vi "Check Range Hi Press.vi"(0 "reference in":refnum<class "Stand.lvclass">, 1 "init":bool, 11 "error in (no error)":errorcluster) -> (4 "reference out":refnum<class "Stand.lvclass">, 15 "error out":errorcluster)   [LabVIEW 2019, in "Stand.lvclass"]
uses:
  Stand.lvclass
  Stand.lvclass/Stand.ctl
  AI_class/AI.lvclass/AI.ctl
  AnalogComparator_class/AnalogComparator.lvclass/AnalogComparator.ctl
  TypeDef/ExecuteStepState.ctl
  AnalogComparator_class/GetStatus.vi
  AI_class/AI.lvclass
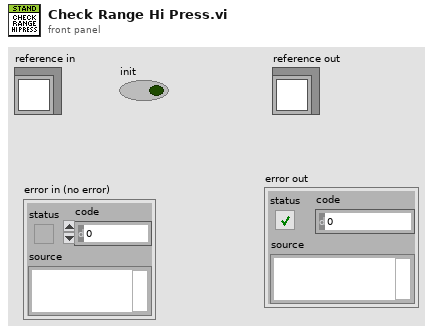
[diagram p1: front panel]
types:
  T1 = typedef "Direction.ctl" = enum8{"DUT", "Chamber"}
  T2 = typedef "AI_Data.ctl" = cluster{"Stat Data":T3, "OutOfRangeMax":bool, "OutOfRangeMin":bool, "HIHI":bool, "HI":bool, "LO":bool, "LOLO":bool}
  T3 = typedef "AI Statistics Data.ctl" = cluster{"raw mean":dbl, "scl mean":dbl, "raw mean 1Hz":dbl, "scl mean 1Hz":dbl}
  T4 = typedef "ExecuteStepState.ctl" = enum16{"Init", "Set: Backpressure ", "Preload: HI", "Set: HI", "Maintenance: HI", "Down: Pressure", "BLOCK"}
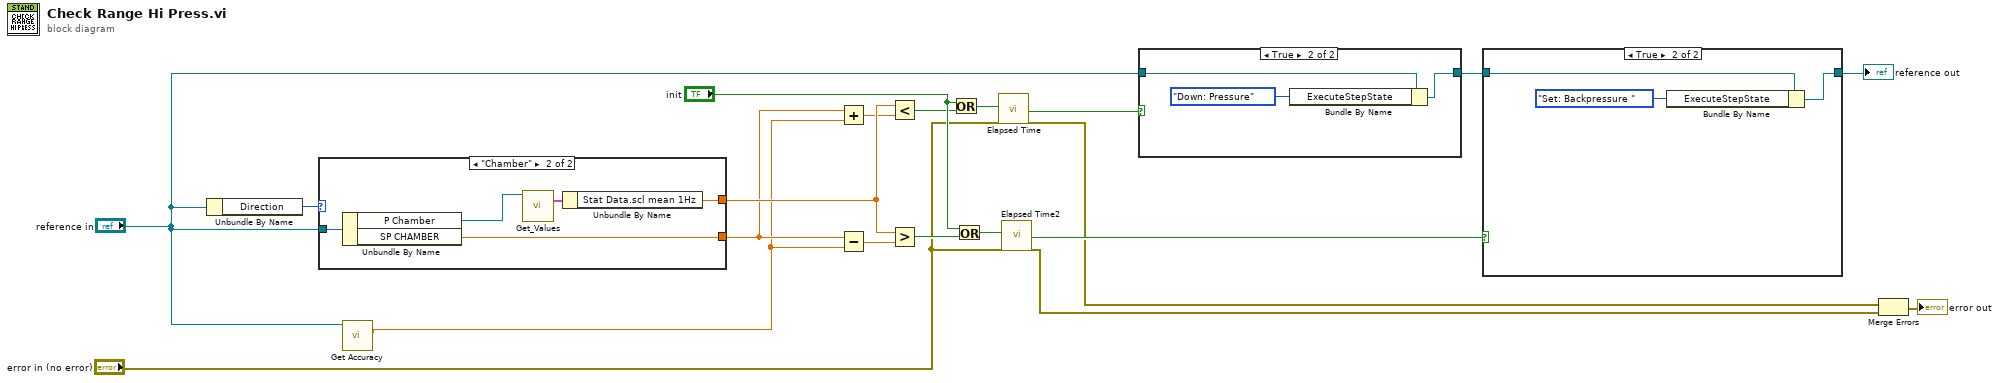
[diagram p0: block diagram]
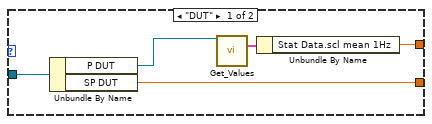
[diagram p4: hidden frame]
diagram:
  n1 = Unbundle By Name("reference in") -> ("Direction"=w7:T1)
  n2 = case shown="\"Chamber\"" w7 {
    tunnel: "reference in" -> [w25 w30]
    tunnel: [w22 w27] -> w11
    tunnel: [w21 w26] -> w15
    frame "DUT" {
      n3 = Unbundle By Name(w25) -> ("P DUT"=w23:refnum<class "AI.lvclass">, "SP DUT"=w22:dbl)
      n4 = call "Get_Values.vi"("reference in"=w23) -> ("Data"=w24:T2)  [unwired: 14 in]
      n5 = Unbundle By Name(w24) -> ("Stat Data.scl mean 1Hz"=w21:dbl)
    }
    frame "Chamber" {
      n6 = Unbundle By Name(w30) -> ("P Chamber"=w28:refnum<class "AI.lvclass">, "SP CHAMBER"=w27:dbl)
      n7 = call "Get_Values.vi"("reference in"=w28) -> ("Data"=w29:T2)  [unwired: 14 in]
      n8 = Unbundle By Name(w29) -> ("Stat Data.scl mean 1Hz"=w26:dbl)
    }
  }
  n9 = call "Get Accuracy.vi"("Stand in"="reference in") -> ("Accuracy [MPa]"=w1:dbl)  [unwired: 10 in]
  n10 = Add(x=w11, y=w1) -> (x+y=w8:dbl)
  n11 = Subtract(x=w11, y=w1) -> (x-y=w14:dbl)
  n12 = Less?(x=w15, y=w8) -> (x < y?=w9:bool)
  n13 = Greater?(x=w15, y=w14) -> (0:w13:bool)
  n14 = Or(x="init", y=w9) -> (x .or. y?=w10:bool)
  n15 = Or(x="init", y=w13) -> (x .or. y?=w12:bool)
  n16 = call "Elapsed Time"("Reset"=w10, "error in (no error)"="error in (no error)") -> ("Time has Elapsed"=w19:bool, "error out"=w4:errorcluster)  [unwired: 10 in, 6 out]
  n17 = call "Elapsed Time2"("Reset"=w12, "error in (no error)"="error in (no error)") -> ("Time has Elapsed"=w18:bool, "error out"=w5:errorcluster)  [unwired: 10 in, 6 out]
  n18 = case shown="True" w19 {
    tunnel: "reference in" -> [w31 w34]
    tunnel: [w31 w33] -> w17
    frame False {
    }
    frame True {
      n19 = Bundle By Name(cluster=w34, "ExecuteStepState"=ExecuteStepState."Down: Pressure" ("Data.ExecuteStepState")) -> (w33:refnum<class "Stand.lvclass">)
    }
  }
  n20 = case shown="True" w18 {
    tunnel: w17 -> [w35 w38]
    tunnel: [w35 w37] -> w20
    frame False {
    }
    frame True {
      n21 = Bundle By Name(cluster=w38, "ExecuteStepState"=ExecuteStepState."Set: Backpressure " ("Data.ExecuteStepState")) -> (w37:refnum<class "Stand.lvclass">)
    }
  }
  "reference out" <- w20
  n22 = Merge Errors(w4, w5) -> (→"error out":errorcluster)
